vi "LimitReached.vi"(8 "error in (no error)":errorcluster, 11 "InterferometryUI in":refnum<class "InterferometryUI.lvclass">) -> (0 "error out":errorcluster, 3 "InterferometryUI out":refnum<class "InterferometryUI.lvclass">)   [LabVIEW 2023, in "InterferometryUI.lvlib" / "InterferometryUI.lvclass"]
uses:
  InterferometryUI.lvclass
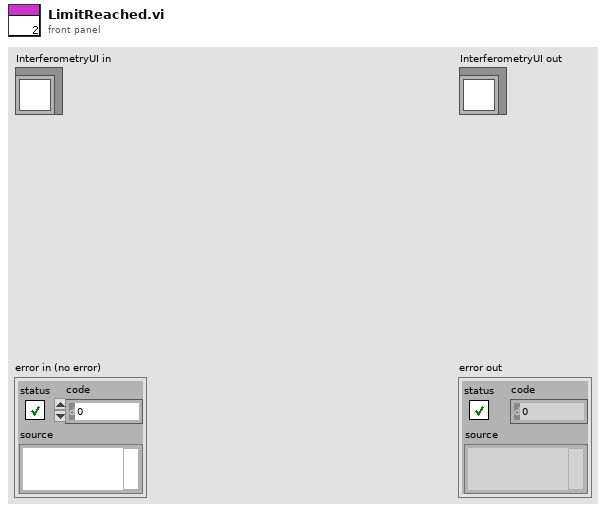
[diagram p1: front panel]
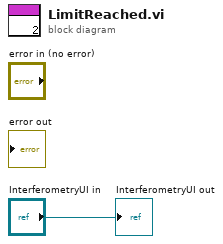
[diagram p0: block diagram]
diagram:
  "InterferometryUI out" <- "InterferometryUI in"
